vi "Fail Result.vi"(8 "error in (no error)":errorcluster) -> (0 "error out":errorcluster)   [LabVIEW 2018]
panel:
  in  "OK":bool
  in  "Stop":bool
  # "FAIL"
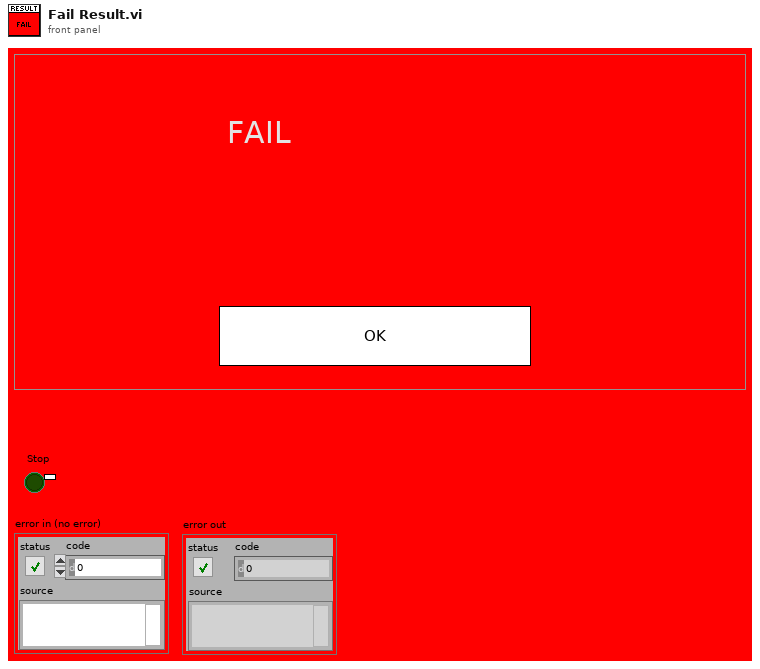
[diagram p1: front panel]
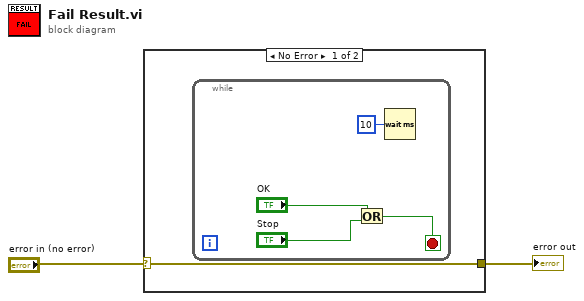
[diagram p0: block diagram]
diagram:
  n1 = case shown="No Error" "error in (no error)" {
    selector: "error in (no error)" -> [w3 w8]
    tunnel: [w3 w8] -> w1
    frame No Error {
      n2 = while {
        stop <- w4 stop-if-true
        n3 = Or(x="OK", y="Stop") -> (x .or. y?=w4:bool)
        n4 = Wait (ms)(milliseconds to wait=u32 10) -> ()  [unwired: 1 out]
      }
    }
    frame Error {
    }
  }
  "error out" <- w1
